vi "Derivative of Pts.vi"(10 "fix first pt?":bool, 11 "pts":cluster{sgl, sgl}[](array[cluster])) -> (3 "pts out":cluster{sgl, sgl}[](array[cluster]))   [LabVIEW 2025]
uses:
  <vilib>/Analysis/NI_AALPro.lvlib
  <vilib>/ptbypt/NI_PtbyPt.lvlib
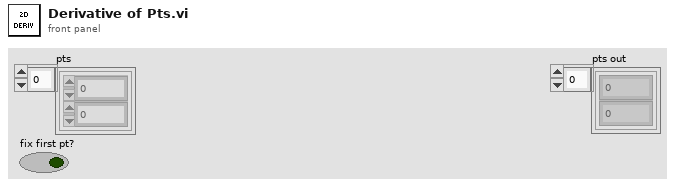
[diagram p1: front panel]
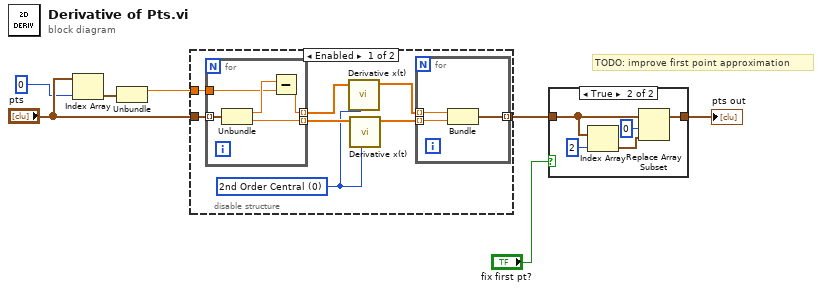
[diagram p0: block diagram]
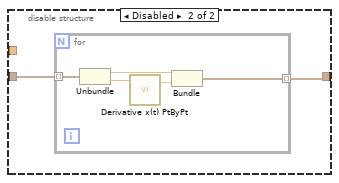
[diagram p3: hidden frame]
diagram:
  # "TODO: improve first point approximation"
  n1 = Index Array(array="pts", index=0) -> (element=w2:cluster{sgl, sgl})
  n2 = Unbundle(w2) -> (w1:sgl)  [unwired: 1 out]
  n3 = disable-structure shown="Enabled" {
    disable-tunnel: "pts" -> [w15 w25]
    disable-tunnel: [w12 w24] -> w7
    disable-tunnel: w1 -> [w11 _]
    frame Enabled {
      w8 = u16 0 items=["2nd Order Central", "4th Order Central", "Forward", "Backward"] ("method")
      n4 = for {
        tunnel: w15 -> [w23] mode=indexing
        tunnel: [w19] -> w10 mode=indexing
        tunnel: [w22] -> w14 mode=indexing
        tunnel: w11 -> [w20]
        n5 = Unbundle(w23) -> (w21:sgl, w22:sgl)
        n6 = Subtract(x=w21, y=w20) -> (x-y=w19:sgl)
      }
      n7 = call <vilib>:"Derivative x(t).vi"("method"=w8, "X"=w10) -> ("dX/dt"=w9:dbl[])  [unwired: 8 in, 1 out]
      n8 = call <vilib>:"Derivative x(t).vi"("method"=w8, "X"=w14) -> ("dX/dt"=w13:dbl[])  [unwired: 8 in, 1 out]
      n9 = for {
        tunnel: w13 -> [w17] mode=indexing
        tunnel: w9 -> [w18] mode=indexing
        tunnel: [w16] -> w12 mode=indexing
        n10 = Bundle(w18, w17) -> (w16:cluster{dbl, dbl})  [unwired: 1 in]
      }
    }
    frame Disabled {
      n11 = for {
        tunnel: w25 -> [w30] mode=indexing
        tunnel: [w26] -> w24 mode=indexing
        n12 = Unbundle(w30) -> (w27:sgl, w29:sgl)
        n13 = call <vilib>:"Derivative x(t) PtByPt.vi"("x"=w29) -> ("dx/dt"=w28:dbl)  [unwired: 3 in, 1 out]
        n14 = Bundle(w27, "dx/dt"=w28) -> (w26:cluster{sgl, "dx/dt":dbl})  [unwired: 1 in]
      }
    }
  }
  n15 = case shown="True" "fix first pt?" {
    tunnel: w7 -> [w31 w36]
    tunnel: [w31 w35] -> w6
    frame False {
    }
    frame True {
      n16 = Index Array(array=w36, index=2) -> (element=w33:cluster{dbl, dbl})
      n17 = Replace Array Subset(array=w36, new element=w33, index=0) -> (w35:cluster{dbl, dbl}[])
    }
  }
  "pts out" <- w6
